vi "GetAlignmentElements.vi"(8 "error in (no error)":errorcluster, 11 "Alignment in":refnum<class "Alignment.lvclass">) -> (0 "error out":errorcluster, 2 "Alignments":T1[](array[typedef]), 3 "Alignment out":refnum<class "Alignment.lvclass">)   [LabVIEW 2021, in "LvMarkdown.lvlib" / "Alignment.lvclass"]
uses:
  Alignment.lvclass
  Alignment.lvclass/Alignment.ctl
  AlignmentEnum.ctl
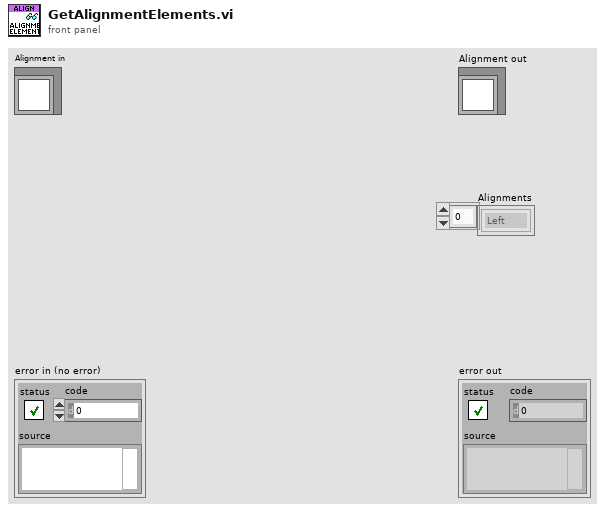
[diagram p1: front panel]
types:
  T1 = typedef "LvMarkdown.lvlib/Alignment.lvclass/AlignmentEnum.ctl" = enum16{"Left", "Center", "Right"}
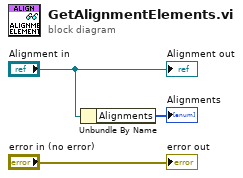
[diagram p0: block diagram]
diagram:
  n1 = Unbundle By Name("Alignment in") -> ("Alignments"=→"Alignments":T1[])
  "error out" <- "error in (no error)"
  "Alignment out" <- "Alignment in"
